vi "Configure Optimum Attenuator for Mixer IMD.vi"(7 "Use Eletronic Attenuator (F)":bool, 8 "error in (no error)":errorcluster, 9 "Frequency offset between F1 and F2":dbl, 10 "Power Level at SA":dbl, 11 "SA-ESA in":refnum<class "SA-ESA.lvclass">) -> (0 "error out":errorcluster, 3 "SA-ESA out":refnum<class "SA-ESA.lvclass">)   [LabVIEW 2020, in "SA-ESA.lvclass"]
uses:
  SA-ESA.lvclass
  C:/Sandbox/RF Bench/Source Code/WiSpry Test Framework/Instruments/Spectrum Analyzer/Spectrum Analyzer.lvclass
  Spectrum Analyzer.lvclass/Spectrum Analyzer.ctl
  Spectrum Analyzer.lvclass
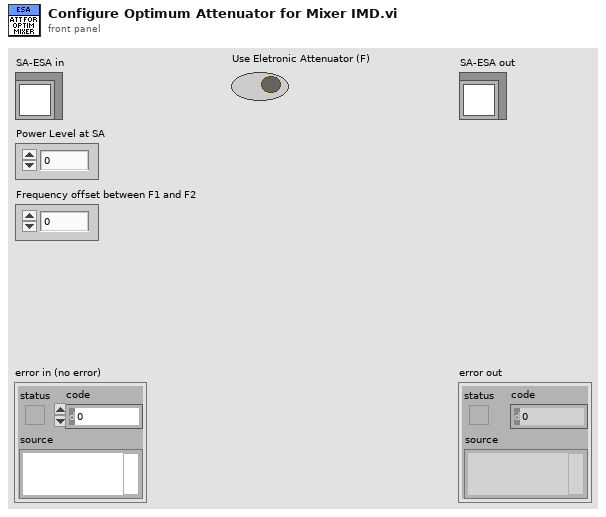
[diagram p1: front panel]
types:
  T1 = cluster{"Offset Frequency":dbl, "Mixer Level":dbl}[]
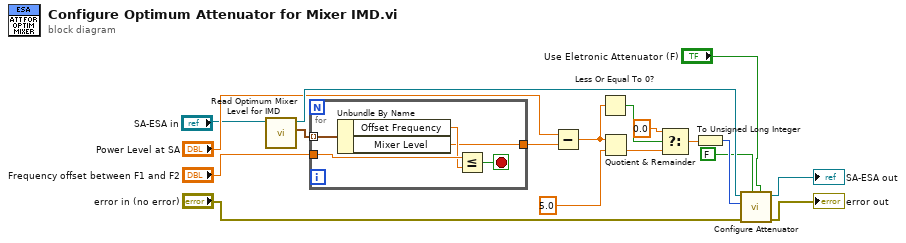
[diagram p0: block diagram]
diagram:
  n1 = call "Read Optimum Mixer Level for IMD.vi"("Spectrum Analyzer in"="SA-ESA in") -> ("Optimum Mixer Level for IMD"=w18:T1, "Spectrum Analyzer out"=w12:refnum<class "SA-ESA.lvclass">)  [unwired: 9 in]
  n2 = for {
    tunnel: w18 -> [w23] mode=indexing
    tunnel: "Frequency offset between F1 and F2" -> [w22]
    tunnel: [w19] -> w17
    stop <- w20 stop-if-true
    n3 = Unbundle By Name(w23) -> ("Offset Frequency"=w21:dbl, "Mixer Level"=w19:dbl)
    n4 = Less Or Equal?(x=w22, y=w21) -> (x <= y?=w20:bool)
  }
  n5 = Subtract(x="Power Level at SA", y=w17) -> (x-y=w14:dbl)
  n6 = Less Or Equal To 0?(x=w14) -> (x <= 0?=w16:bool)
  n7 = Quotient & Remainder(x=w14, y=5.0 ("f")) -> (floor(x/y)=w13:dbl)  [unwired: 1 out]
  n8 = Select(t=0.0, s=w16, f=w13) -> (s? t:f=w11:dbl)
  n9 = To Unsigned Long Integer(number=w11) -> (unsigned 32bit integer=w10:u32)
  n10 = call-dynamic "Configure Attenuator.vi"("Use Eletronic Attenuator (F)"="Use Eletronic Attenuator (F)", "Auto Attenuator (T)"=FALSE, "error in (no error)"="error in (no error)", "Attenuator (dB)"=w10, "SA-ESA in"=w12) -> ("error out"=→"error out":errorcluster, "SA-ESA out"=→"SA-ESA out":refnum<class "SA-ESA.lvclass">)  [unwired: 5 in]
